vi "calculator.vi"() -> ()   [LabVIEW 2010]
panel:
  in  "equals":bool
  in  "stop":bool
  in  "Display":dbl format="%#_20g"
  in  "divide":bool
  in  "add":bool
  in  "subtract":bool
  in  "multiply":bool
  in  "0":bool
  in  "dec":bool
  in  "9":bool
  in  "8":bool
  in  "7":bool
  in  "6":bool
  in  "5":bool
  in  "4":bool
  in  "3":bool
  in  "2":bool
  in  "1":bool
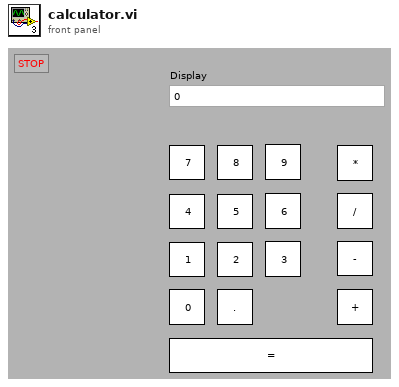
[diagram p1: front panel]
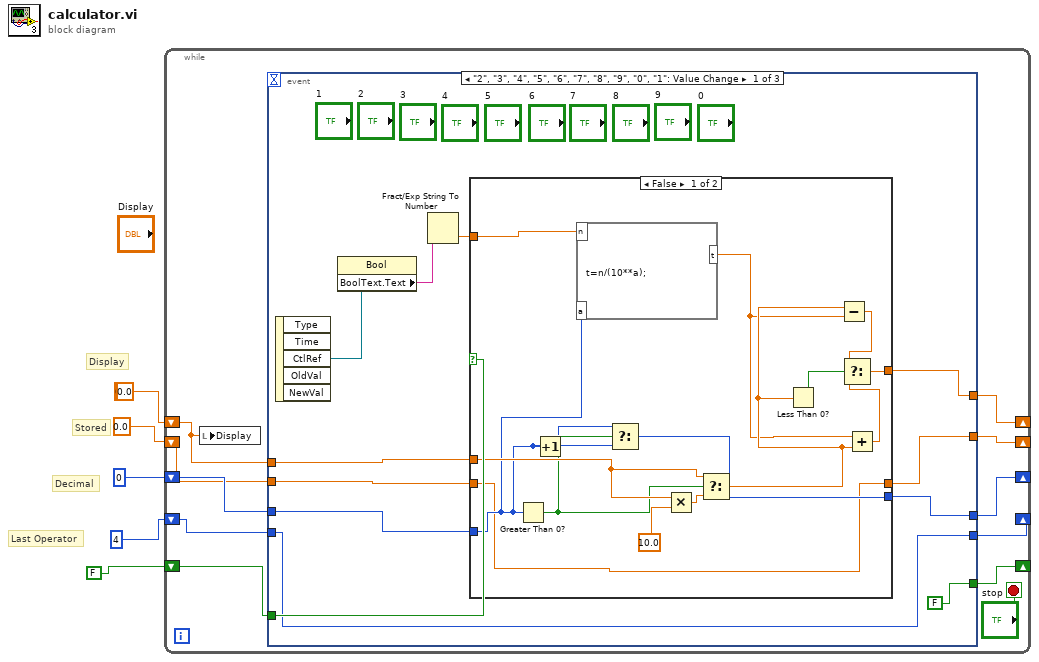
[diagram p0: block diagram]
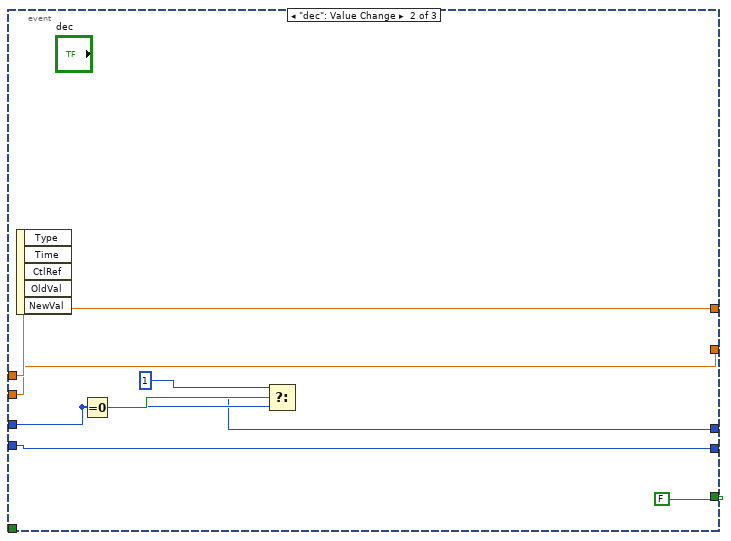
[diagram p3: hidden frame]
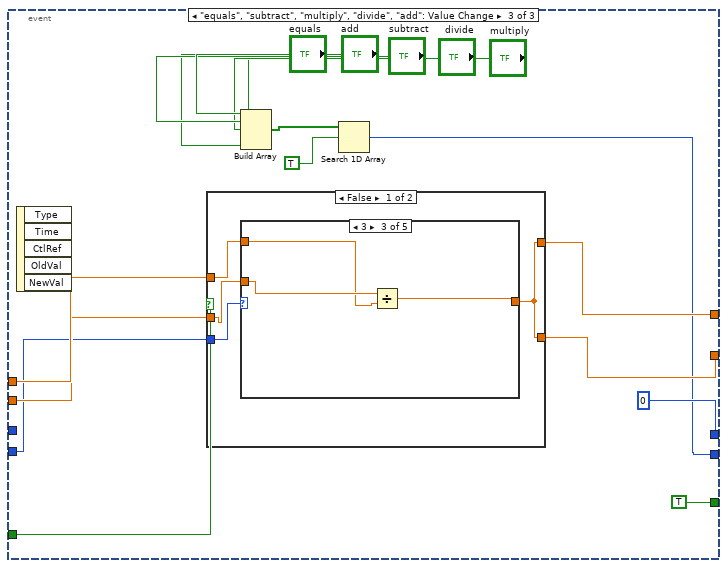
[diagram p4: hidden frame]
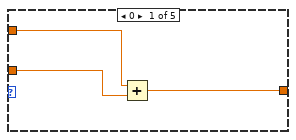
[diagram p5: hidden frame]
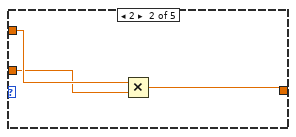
[diagram p6: hidden frame]
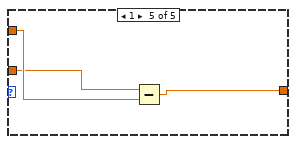
[diagram p8: hidden frame]
diagram:
  (unwired) 0.0
  # "Stored"
  # "Decimal"
  # "Last Operator"
  # "Display"
  n1 = while {
    shift-right: [w14] -> _
    shift-left: 0.0 -> [w15]
    shift-right: [w13] -> _
    shift-left: 0 ("dec") -> [w12]
    shift-right: [w11] -> _
    shift-left: 4 -> [w9]
    shift-right: [w8] -> _
    shift-left: FALSE -> [w7]
    shift-right: [w6] -> _
    shift-left: 0.0 -> [w10]
    stop <- "stop" stop-if-true
    n2 = local write "Display"(w15) -> ()
    n3 = event shown="[0] \"2\", \"3\", \"4\", \"5\", \"6\", \"7\", \"8\", \"9\", \"0\", \"1\": Value Change" {
      selector: _ -> [_ _ _]
      dyn-events: _ -> [_ _ _]
      timeout: _ -> [_ _ _]
      tunnel: w15 -> [w25 w54 w70]
      tunnel: [w26 w54 w64] -> w14
      tunnel: w12 -> [w23 w52 _]
      tunnel: [w24 w50 0] -> w13
      tunnel: [w18 w49 w55] -> w11
      tunnel: w10 -> [w21 w47 w69]
      tunnel: w9 -> [w18 w49 w68]
      tunnel: [FALSE FALSE TRUE] -> w8
      tunnel: w7 -> [w20 _ w65]
      tunnel: [w19 w47 w63] -> w6
      event "2", "3", "4", "5", "6", "7", "8", "9", "0", "1": Value Change {
        n4 = event-data() -> ("CtlRef"=w28:refnum<vi>)  [unwired: 1 in, 4 out]
        n5 = property class="Bool"(reference=w28) -> ("BoolText.Text"=w27:string)  [unwired: 1 in, 2 out]
        n6 = Fract/Exp String To Number(string=w27) -> (number=w17:dbl)  [unwired: 3 in, 1 out]
        n7 = case shown="False" w20 {
          tunnel: [w39 w46] -> w26
          tunnel: w25 -> [w38 w44]
          tunnel: w17 -> [w35 w46]
          tunnel: [w32 w45] -> w24
          tunnel: w23 -> [w30 w45]
          tunnel: [w29 w44] -> w19
          tunnel: w21 -> [w29 _]
          frame False {
            n8 = Greater Than 0?(x=w30) -> (x > 0?=w34:bool)
            n9 = Increment(x=w30) -> (x+1=w33:i32)
            n10 = formula code="t=n/(10**a);"("n"=w35, "a"=w30) -> ("t"=w31:dbl)
            n11 = Select(t=w33, s=w34, f=w30) -> (s? t:f=w32:i32)
            n12 = Multiply(x=w38, y=10.0) -> (x*y=w37:dbl)
            n13 = Select(t=w38, s=w34, f=w37) -> (s? t:f=w36:dbl)
            n14 = Less Than 0?(x=w36) -> (x < 0?=w42:bool)
            n15 = Subtract(x=w36, y=w31) -> (x-y=w40:dbl)
            n16 = Add(x=w31, y=w36) -> (x+y=w41:dbl)
            n17 = Select(t=w40, s=w42, f=w41) -> (s? t:f=w39:dbl)
          }
          frame True {
          }
        }
      }
      event "dec": Value Change {
        n18 = event-data() -> ()  [unwired: 1 in, 5 out]
        n19 = Equal To 0?(x=w52) -> (x = 0?=w53:bool)
        n20 = Select(t=1, s=w53, f=w52) -> (s? t:f=w50:i32)
      }
      event "equals", "subtract", "multiply", "divide", "add": Value Change {
        n21 = event-data() -> ()  [unwired: 1 in, 5 out]
        n22 = case shown="False" w65 {
          tunnel: w70 -> [w74 w89]
          tunnel: w69 -> [w72 w88]
          tunnel: w68 -> [w73 _]
          tunnel: [w71 w88] -> w63
          tunnel: [w71 w89] -> w64
          frame False {
            n23 = case shown="3" w73 {
              tunnel: w74 -> [w77 w80 w82 w84 w87]
              tunnel: w72 -> [w76 w79 w83 _ w86]
              tunnel: [w75 w78 w81 w84 w85] -> w71
              frame 0 {
                n24 = Add(x=w77, y=w76) -> (x+y=w75:dbl)
              }
              frame 2 {
                n25 = Multiply(x=w80, y=w79) -> (x*y=w78:dbl)
              }
              frame 3 {
                n26 = Divide(x=w83, y=w82) -> (x/y=w81:dbl)
              }
              frame 4, Default {
              }
              frame 1 {
                n27 = Subtract(x=w86, y=w87) -> (x-y=w85:dbl)
              }
            }
          }
          frame True {
          }
        }
        n28 = Build Array("add", "subtract", "multiply", "divide", "equals") -> (w60:bool[])
        n29 = Search 1D Array(1D array=w60, element=TRUE) -> (index of element=w55:i32)  [unwired: 1 in]
      }
    }
  }
